vi "Send Request, JSON Payload.vi"(0 "IPEndPoint":T1, 7 "Message":string, 9 "Payload":string="{}", 11 "error in (no error)":errorcluster) -> (4 "IPEndPoint thru":T1, 6 "Code":i32, 8 "Command":string, 10 "Payload":string, 15 "error out":errorcluster)   [LabVIEW 2020, in "epl-network.lvlib"]
uses:
  epl-network.lvlib
  Typedefs/IPEndPoint.ctl
  Typedefs/TCP Message.ctl
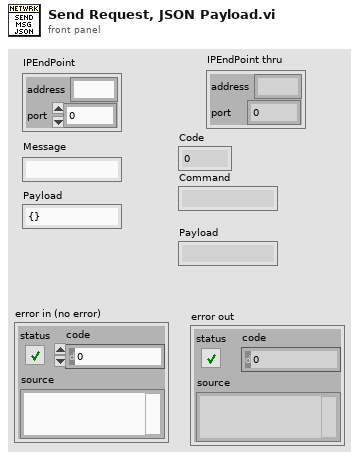
[diagram p1: front panel]
types:
  T1 = typedef "epl-network.lvlib/IPEndPoint.ctl" = cluster{"address":string, "port":i32}
  T2 = typedef "epl-network.lvlib/TCP Message.ctl" = cluster{"Code":i32, "Command":string, "Payload":string}
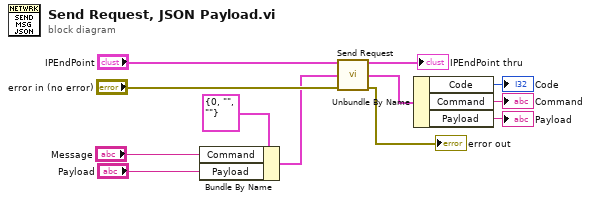
[diagram p0: block diagram]
diagram:
  n1 = Bundle By Name(cluster=T2 {"Code"=0, "Command"="", "Payload"=""} ("TCPMessage"), "Command"="Message", "Payload"="Payload") -> (w8:T2)
  n2 = call "Send Request.vi"("IPEndPoint"="IPEndPoint", "TCPMessage"=w8, "error in (no error)"="error in (no error)") -> ("IPEndPoint thru"=→"IPEndPoint thru":T1, "Response"=w4:T2, "error out"=→"error out":errorcluster)  [unwired: 10 in]
  n3 = Unbundle By Name(w4) -> ("Code"=→"Code":i32, "Command"=→"Command":string, "Payload"=→"Payload":string)
